vi "grSim Robot Command.vi"(9 "Array In":u8[](array[numeric]), 11 "Robot":T1 {"Vel Esquerda 3" format="%1_6f"; "Vel Esquerda 2" format="%1_6f"; "Vel Esquerda 1" format="%1_6f"; "Vel Direita 3" format="%1_6f"; "Vel Direita 2" format="%1_6f"; "Vel Direita 1" format="%1_6f"}) -> (1 "Array":u8[](array[numeric]))   [LabVIEW 2017]
uses:
  Viewer Robot Command.ctl
panel:
  in  "input cluster":T1 {"Vel Esquerda 3" format="%1_6f"; "Vel Esquerda 2" format="%1_6f"; "Vel Esquerda 1" format="%1_6f"; "Vel Direita 3" format="%1_6f"; "Vel Direita 2" format="%1_6f"; "Vel Direita 1" format="%1_6f"}
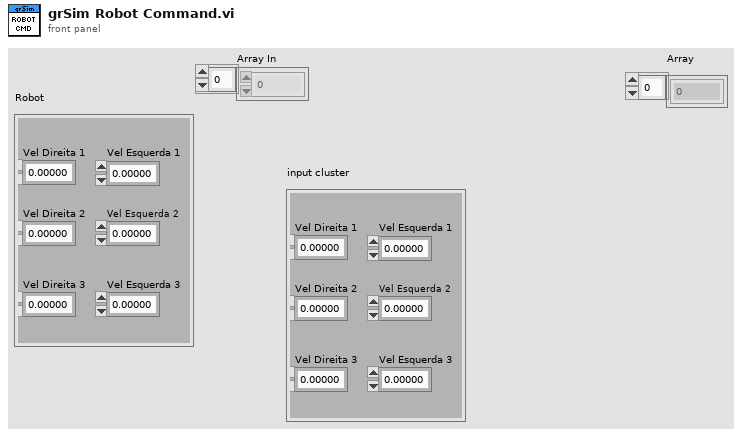
[diagram p1: front panel]
types:
  T1 = typedef "Viewer Robot Command.ctl" = cluster{"Vel Direita 1\n":dbl, "Vel Direita 2":dbl, "Vel Direita 3":dbl, "Vel Esquerda 1\n":dbl, "Vel Esquerda 2":dbl, "Vel Esquerda 3":dbl}
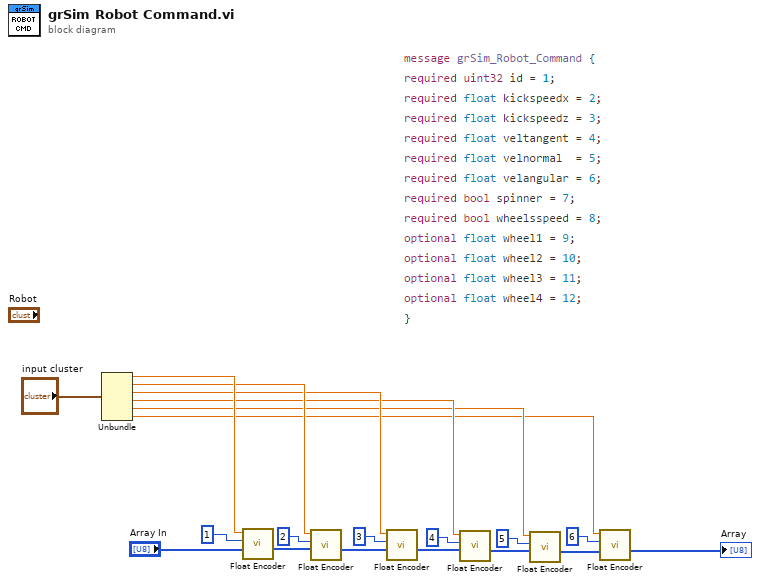
[diagram p0: block diagram]
diagram:
  n1 = Unbundle("input cluster") -> ("Vel Direita 1"=w7:dbl, "Vel Direita 2"=w5:dbl, "Vel Direita 3"=w4:dbl, "Vel Esquerda 1"=w3:dbl, "Vel Esquerda 2"=w2:dbl, "Vel Esquerda 3"=w1:dbl)
  n2 = call "Float Encoder.vi"("Array In"="Array In", "Key"=u32 1, "Value"=w7) -> ("Array"=w9:u8[])  [unwired: 8 in]
  n3 = call "Float Encoder.vi"("Array In"=w9, "Key"=u32 2, "Value"=w5) -> ("Array"=w15:u8[])  [unwired: 8 in]
  n4 = call "Float Encoder.vi"("Array In"=w15, "Key"=u32 3, "Value"=w4) -> ("Array"=w14:u8[])  [unwired: 8 in]
  n5 = call "Float Encoder.vi"("Array In"=w14, "Key"=u32 4, "Value"=w3) -> ("Array"=w13:u8[])  [unwired: 8 in]
  n6 = call "Float Encoder.vi"("Array In"=w13, "Key"=u32 5, "Value"=w2) -> ("Array"=w12:u8[])  [unwired: 8 in]
  n7 = call "Float Encoder.vi"("Array In"=w12, "Key"=u32 6, "Value"=w1) -> ("Array"=→"Array":u8[])  [unwired: 8 in]
